vi "Prop Controller 4.vi"(10 "GIC Input":T1={"Real/Sim"=FALSE, "WP Lats and Longs"={"WP Lats"=[37.152345, 37.152256, 37.152877, 37.152903, 37.152565, 37.152792, 37.152806, 37.152779, 37.152868, 37.152484], "WP Longs"=[81.267743, 81.267312, 81.267112, 81.267332, 81.267916, 81.267137, 81.267874, 81.267301, 81.267913, 81.26772]}, "GPS Time Int"=2.4, "GPS Com Port"="COM4", "Compass Com Port"="COM6", "Prop Com Port"="COM6", "GPS Data"=[37.1526, 81.2675, 7.3], "Compass"=0.0, "LMS Vector"=array[961 elements], "Vision Vector"=[], "Direction Cmd"=270.0, "Speed Cmd"=0.0, "Time of Last GPS"=0.0, "WP Vector"=[-142.7829201595333, 34.51991008972894], "WP Number"=1, "Num of WPs"=10, "SW Map"=array80x80[6400 elements], "Obst Lats and Longs"={"Obst Lats"=[37.1524, 37.152256, 37.152877, 37.152903, 37.152565, 37.152792, 37.152806, 37.152779, 37.152868, 37.152484], "Obst Longs"=[81.2678, 81.267312, 81.267112, 81.267332, 81.267916, 81.267137, 81.267874, 81.267301, 81.267913, 81.26772]}, "Parameters"=[3.0, 0.0, 0.0, 0.0, 50.0, 0.0, 40.0, 65.0, 40.0, 60.0, 5.0, 0.0, 37.1526, 81.2675, 7.3, 1.0, 0.0, 15.0], "Path Cluster"={"Path x nodes"=[40.0, 40.0, 40.0, 40.0, 40.0, 40.0, 0.0, 0.0, 0.0, 0.0, 0.0, 0.0, 0.0, 0.0, 0.0, 0.0, 0.0, 0.0, 0.0, 0.0, 0.0, 0.0, 0.0, 0.0, 0.0, 0.0, 0.0, 0.0, 0.0, 0.0, 0.0, 0.0, 0.0, 0.0, 0.0, 0.0, 0.0, 0.0, 0.0, 0.0, 0.0, 0.0, 0.0, 0.0, 0.0, 0.0, 0.0, 0.0, 0.0, 0.0, 0.0, 0.0, 0.0, 0.0, 0.0, 0.0, 0.0, 0.0, 0.0, 0.0, 0.0, 0.0, 0.0, 0.0, 0.0, 0.0, 0.0, 0.0, 0.0, 0.0, 0.0, 0.0, 0.0, 0.0, 0.0, 0.0, 0.0, 0.0, 0.0, 0.0, 0.0, 0.0, 0.0, 0.0, 0.0, 0.0, 0.0, 0.0, 0.0, 0.0, 0.0, 0.0, 0.0, 0.0, 0.0, 0.0, 0.0, 0.0, 0.0, 0.0, 0.0, 0.0, 0.0, 0.0, 0.0, 0.0, 0.0, 0.0, 0.0, 0.0, 0.0, 0.0, 0.0, 0.0, 0.0, 0.0, 0.0, 0.0, 0.0, 0.0, 0.0, 0.0, 0.0, 0.0, 0.0, 0.0, 0.0, 0.0, 0.0, 0.0, 0.0, 0.0, 0.0, 0.0, 0.0, 0.0, 0.0, 0.0, 0.0, 0.0, 0.0, 0.0, 0.0, 0.0, 0.0, 0.0, 0.0, 0.0, 0.0, 0.0, 0.0, 0.0, 0.0, 0.0, 0.0, 0.0, 0.0, 0.0, 0.0, 0.0, 0.0, 0.0, 0.0, 0.0, 0.0, 0.0, 0.0, 0.0, 0.0, 0.0, 0.0, 0.0, 0.0, 0.0, 0.0, 0.0, 0.0, 0.0, 0.0, 0.0, 0.0, 0.0, 0.0, 0.0, 0.0, 0.0, 0.0, 0.0, 0.0, 0.0, 0.0, 0.0, 0.0, 0.0, 0.0, 0.0, 0.0, 0.0, 0.0, 0.0, 0.0, 0.0, 0.0, 0.0, 0.0, 0.0, 0.0, 0.0, 0.0, 0.0, 0.0, 0.0, 0.0, 0.0, 0.0, 0.0, 0.0, 0.0, 0.0, 0.0, 0.0, 0.0, 0.0, 0.0, 0.0, 0.0, 0.0, 0.0, 0.0, 0.0, 0.0, 0.0, 0.0, 0.0, 0.0, 0.0, 0.0, 0.0, 0.0, 0.0, 0.0, 0.0, 0.0, 0.0, 0.0, 0.0, 0.0, 0.0, 0.0, 0.0, 0.0, 0.0, 0.0, 0.0, 0.0, 0.0, 0.0, 0.0, 0.0, 0.0, 0.0, 0.0, 0.0, 0.0, 0.0, 0.0, 0.0, 0.0, 0.0, 0.0, 0.0, 0.0, 0.0, 0.0, 0.0, 0.0, 0.0, 0.0, 0.0, 0.0, 0.0, 0.0, 0.0, 0.0, 0.0, 0.0, 0.0, 0.0, 0.0, 0.0, 0.0, 0.0, 0.0, 0.0, 0.0, 0.0, 0.0, 0.0, 0.0, 0.0, 0.0, 0.0, 0.0, 0.0, 0.0, 0.0, 0.0, 0.0, 0.0, 0.0, 0.0, 0.0, 0.0, 0.0, 0.0, 0.0, 0.0, 0.0, 0.0, 0.0], "Path y nodes"=[60.0, 61.0, 62.0, 63.0, 64.0, 65.0, 0.0, 0.0, 0.0, 0.0, 0.0, 0.0, 0.0, 0.0, 0.0, 0.0, 0.0, 0.0, 0.0, 0.0, 0.0, 0.0, 0.0, 0.0, 0.0, 0.0, 0.0, 0.0, 0.0, 0.0, 0.0, 0.0, 0.0, 0.0, 0.0, 0.0, 0.0, 0.0, 0.0, 0.0, 0.0, 0.0, 0.0, 0.0, 0.0, 0.0, 0.0, 0.0, 0.0, 0.0, 0.0, 0.0, 0.0, 0.0, 0.0, 0.0, 0.0, 0.0, 0.0, 0.0, 0.0, 0.0, 0.0, 0.0, 0.0, 0.0, 0.0, 0.0, 0.0, 0.0, 0.0, 0.0, 0.0, 0.0, 0.0, 0.0, 0.0, 0.0, 0.0, 0.0, 0.0, 0.0, 0.0, 0.0, 0.0, 0.0, 0.0, 0.0, 0.0, 0.0, 0.0, 0.0, 0.0, 0.0, 0.0, 0.0, 0.0, 0.0, 0.0, 0.0, 0.0, 0.0, 0.0, 0.0, 0.0, 0.0, 0.0, 0.0, 0.0, 0.0, 0.0, 0.0, 0.0, 0.0, 0.0, 0.0, 0.0, 0.0, 0.0, 0.0, 0.0, 0.0, 0.0, 0.0, 0.0, 0.0, 0.0, 0.0, 0.0, 0.0, 0.0, 0.0, 0.0, 0.0, 0.0, 0.0, 0.0, 0.0, 0.0, 0.0, 0.0, 0.0, 0.0, 0.0, 0.0, 0.0, 0.0, 0.0, 0.0, 0.0, 0.0, 0.0, 0.0, 0.0, 0.0, 0.0, 0.0, 0.0, 0.0, 0.0, 0.0, 0.0, 0.0, 0.0, 0.0, 0.0, 0.0, 0.0, 0.0, 0.0, 0.0, 0.0, 0.0, 0.0, 0.0, 0.0, 0.0, 0.0, 0.0, 0.0, 0.0, 0.0, 0.0, 0.0, 0.0, 0.0, 0.0, 0.0, 0.0, 0.0, 0.0, 0.0, 0.0, 0.0, 0.0, 0.0, 0.0, 0.0, 0.0, 0.0, 0.0, 0.0, 0.0, 0.0, 0.0, 0.0, 0.0, 0.0, 0.0, 0.0, 0.0, 0.0, 0.0, 0.0, 0.0, 0.0, 0.0, 0.0, 0.0, 0.0, 0.0, 0.0, 0.0, 0.0, 0.0, 0.0, 0.0, 0.0, 0.0, 0.0, 0.0, 0.0, 0.0, 0.0, 0.0, 0.0, 0.0, 0.0, 0.0, 0.0, 0.0, 0.0, 0.0, 0.0, 0.0, 0.0, 0.0, 0.0, 0.0, 0.0, 0.0, 0.0, 0.0, 0.0, 0.0, 0.0, 0.0, 0.0, 0.0, 0.0, 0.0, 0.0, 0.0, 0.0, 0.0, 0.0, 0.0, 0.0, 0.0, 0.0, 0.0, 0.0, 0.0, 0.0, 0.0, 0.0, 0.0, 0.0, 0.0, 0.0, 0.0, 0.0, 0.0, 0.0, 0.0, 0.0, 0.0, 0.0, 0.0, 0.0, 0.0, 0.0, 0.0, 0.0, 0.0, 0.0, 0.0, 0.0, 0.0, 0.0, 0.0, 0.0, 0.0, 0.0, 0.0, 0.0, 0.0, 0.0, 0.0, 0.0, 0.0, 0.0, 0.0, 0.0, 0.0, 0.0, 0.0, 0.0, 0.0, 0.0]}, "     Use ?\nOff       On"=[FALSE, TRUE, FALSE, TRUE]} {"Obst Lats and Longs"."Obst Longs" format="%#_8g"; "Obst Lats and Longs"."Obst Lats" format="%#_8g"}) -> (0 "Prop VISA Resource Name":refnum<visa-resource-name>)   [LabVIEW 2014]
uses:
  <vilib>/Instr/_visa.llb/VISA Configure Serial Port (Instr).vi
panel:
  # "ARES Prop Control   2"
  # "GPS"
  # "LMS"
  # "Vision"
  # "Prop"
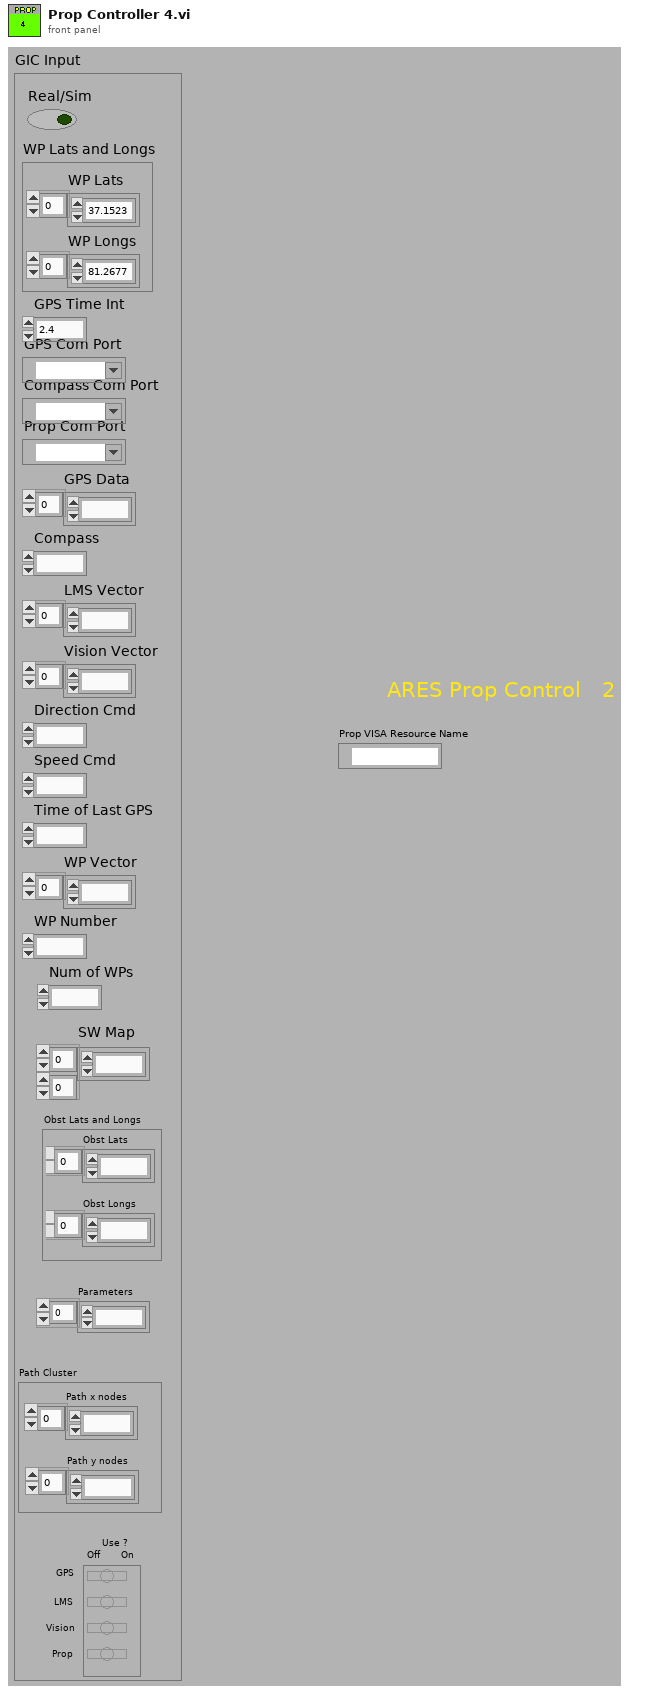
[diagram p1: front panel]
types:
  T1 = cluster{"Real/Sim":bool, "WP Lats and Longs":cluster{"WP Lats":dbl[], "WP Longs":dbl[]}, "GPS Time Int":dbl, "GPS Com Port":refnum<visa-resource-name>, "Compass Com Port":refnum<visa-resource-name>, "Prop Com Port":refnum<visa-resource-name>, "GPS Data":dbl[], "Compass":dbl, "LMS Vector":dbl[], "Vision Vector":dbl[], "Direction Cmd":dbl, "Speed Cmd":dbl, "Time of Last GPS":dbl, "WP Vector":dbl[], "WP Number":i32, "Num of WPs":i16, "SW Map":i32[][], "Obst Lats and Longs":cluster{"Obst Lats":dbl[], "Obst Longs":dbl[]}, "Parameters":dbl[], "Path Cluster":cluster{"Path x nodes":dbl[], "Path y nodes":dbl[]}, "     Use ?\nOff       On":bool[]}
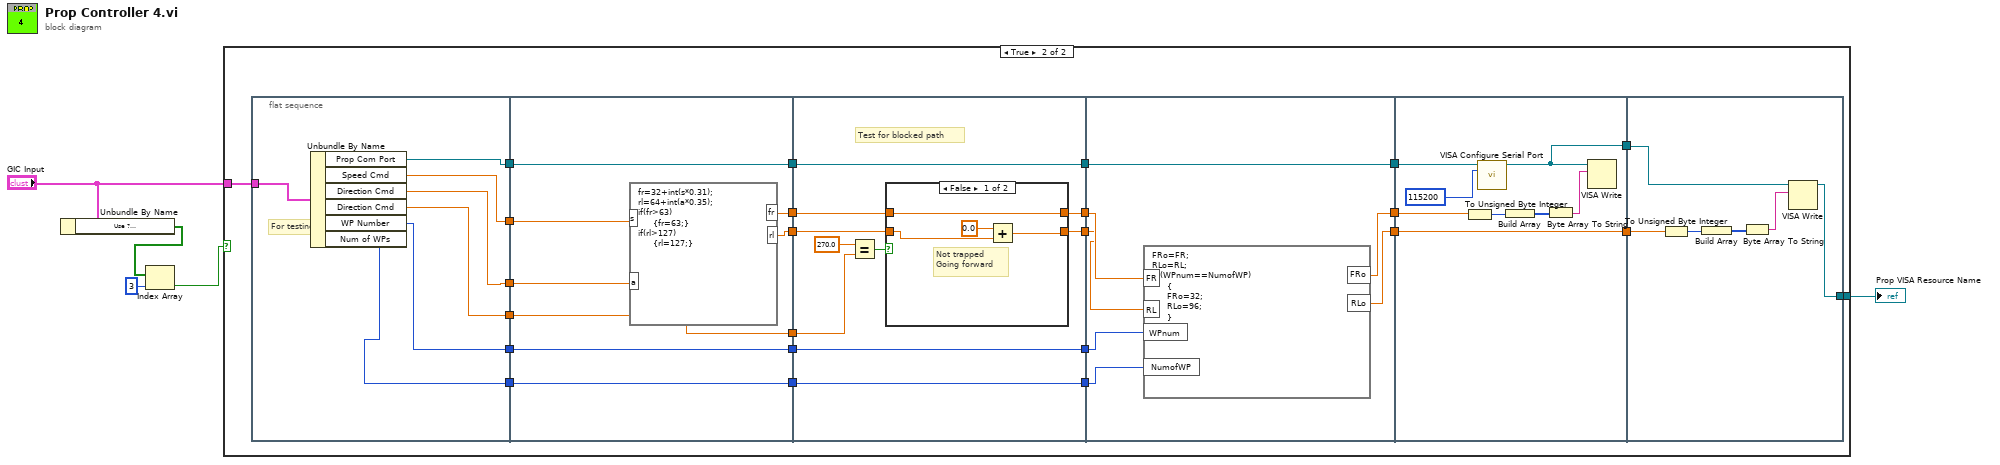
[diagram p0: block diagram]
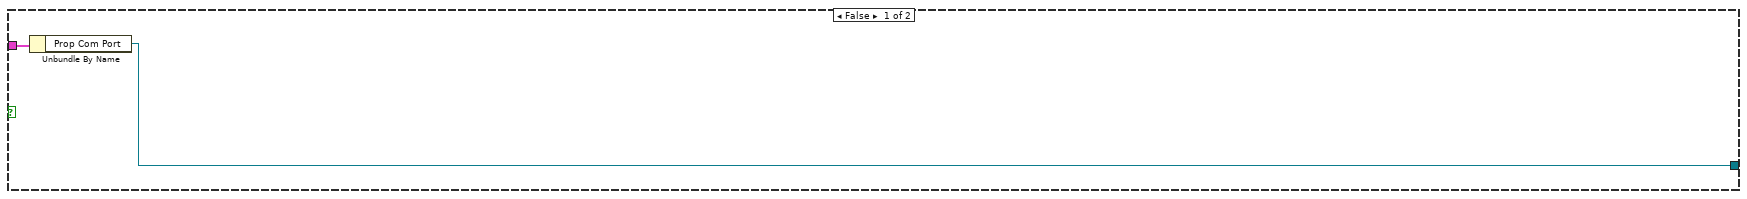
[diagram p2: hidden frame]
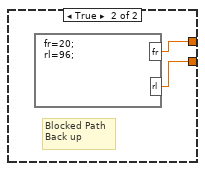
[diagram p3: hidden frame]
diagram:
  n1 = Unbundle By Name("GIC Input") -> ("Use ?\nOff       On"=w4:bool[])
  n2 = Index Array(array=w4, index=3) -> (element=w2:bool)
  n3 = case shown="True" w2 {
    tunnel: "GIC Input" -> [w7 w25]
    tunnel: [w6 w8] -> w1
    frame False {
      n4 = Unbundle By Name(w7) -> ("Prop Com Port"=w6:refnum<visa-resource-name>)
    }
    frame True {
      n5 = flat-sequence {
        tunnel: [w38] -> w24
        tunnel: [w37] -> w23
        tunnel: [w36] -> w22
        tunnel: [w35] -> w21
        tunnel: w25 -> [w34]
        tunnel: [w33] -> w12
        tunnel: [w32] -> w9
        tunnel: [w46] -> w31
        tunnel: [w43] -> w30
        tunnel: [w42] -> w29
        tunnel: [w41] -> w28
        tunnel: w21 -> [w41]
        tunnel: w22 -> [w44]
        tunnel: w23 -> [w45]
        tunnel: w24 -> [w46]
        tunnel: [w40] -> w13
        tunnel: w12 -> [w40]
        tunnel: [w39] -> w10
        tunnel: w9 -> [w39]
        tunnel: w31 -> [w56]
        tunnel: [w56] -> w20
        tunnel: w30 -> [w52]
        tunnel: [w51] -> w18
        tunnel: w29 -> [w50]
        tunnel: [w49] -> w16
        tunnel: w28 -> [w53]
        tunnel: [w48] -> w14
        tunnel: w13 -> [w48]
        tunnel: [w47] -> w11
        tunnel: w10 -> [w47]
        tunnel: w20 -> [w69]
        tunnel: [w69] -> w19
        tunnel: w18 -> [w68]
        tunnel: [w66] -> w17
        tunnel: w16 -> [w67]
        tunnel: [w65] -> w15
        tunnel: w14 -> [w64]
        tunnel: w11 -> [w63]
        tunnel: [w73] -> w27
        tunnel: w19 -> [w72]
        tunnel: w17 -> [w71]
        tunnel: [w70] -> w26
        tunnel: w15 -> [w70]
        tunnel: w27 -> [w80]
        tunnel: w26 -> [w79]
        tunnel: [w78] -> w8
        frame #0 {
          # "For testing:"
          n6 = Unbundle By Name(w34) -> ("Prop Com Port"=w38:refnum<visa-resource-name>, "Speed Cmd"=w37:dbl, "Direction Cmd"=w36:dbl, "Direction Cmd"=w35:dbl, "WP Number"=w33:i32, "Num of WPs"=w32:i16)
        }
        frame #1 {
          n7 = formula code="fr=32+int(s*0.31);\nrl=64+int(a*0.35);\nif(fr>63)\n     {fr=63;}\nif(rl>127)\n     {rl=127;}"("s"=w45, "a"=w44) -> ("fr"=w43:dbl, "rl"=w42:dbl)
        }
        frame #2 {
          # "Test for blocked path"
          n8 = Equal?(x=270.0, y=w53) -> (x = y?=w55:bool)
          n9 = case shown="False" w55 {
            tunnel: w52 -> [w60 _]
            tunnel: [w60 w62] -> w51
            tunnel: w50 -> [w58 _]
            tunnel: [w59 w61] -> w49
            frame False {
              # "Not trapped\nGoing forward"
              n10 = Add(x=0.0, y=w58) -> (x+y=w59:dbl)
            }
            frame True {
              # "Blocked Path\nBack up"
              n11 = formula code="fr=20;\nrl=96;"() -> ("fr"=w62:dbl, "rl"=w61:dbl)
            }
          }
        }
        frame #3 {
          n12 = formula code="FRo=FR;\nRLo=RL;\nif (WPnum==NumofWP)\n     {\n     FRo=32;\n     RLo=96;\n     }"("FR"=w68, "RL"=w67, "WPnum"=w64, "NumofWP"=w63) -> ("FRo"=w66:dbl, "RLo"=w65:dbl)
        }
        frame #4 {
          n13 = To Unsigned Byte Integer(number=w71) -> (unsigned 8bit integer=w75:u8)
          n14 = call-poly "VISA Configure Serial Port"("VISA resource name"=w72, "baud rate (9600)"=115200) -> ("VISA resource name out"=w73:refnum<visa-resource-name>)  [unwired: 12 in, 1 out]
          n15 = Build Array(w75) -> (w74:u8[])
          n16 = Byte Array To String(unsigned byte array=w74) -> (string=w76:string)
          n17 = VISA Write(VISA resource name=w73, write buffer=w76) -> ()  [unwired: 1 in, 3 out]
        }
        frame #5 {
          n18 = To Unsigned Byte Integer(number=w79) -> (unsigned 8bit integer=w82:u8)
          n19 = Build Array(w82) -> (w83:u8[])
          n20 = Byte Array To String(unsigned byte array=w83) -> (string=w81:string)
          n21 = VISA Write(VISA resource name=w80, write buffer=w81) -> (VISA resource name out=w78:refnum<visa-resource-name>)  [unwired: 1 in, 2 out]
        }
      }
    }
  }
  "Prop VISA Resource Name" <- w1
